vi "Set_coordenadas_estacion.vi"(8 "error in (no error)":errorcluster, 10 "MODO":T1=enum."CONFIG ESTACION", 11 "VISA SESSION":refnum<visa-resource-name>) -> (0 "error out":errorcluster, 3 "Coordenadas_estacion 2":T2)   [LabVIEW 2019]
uses:
  Type_defs/Coordenadas_estacion.ctl
  Type_defs/state_coordenadas.ctl
  LABVIEW_ROBOT_MASTER/Type_defs/TAREAS_ROBOT.ctl
  <vilib>/Utility/error.llb/Error Cluster From Error Code.vi
  <vilib>/ErrorRing/Error Ring.xnode
panel:
  in  "Tab Control":enum32{"Page 1", "Page 2"}(tab)
  in  "EXIT":bool
  in  "CONTINUAR":bool
  in  "Set coordenadas bandejas":bool
  out "COORDENADAS ESTACION DE TRABAJO":T2
  out "Estado FSM":T3
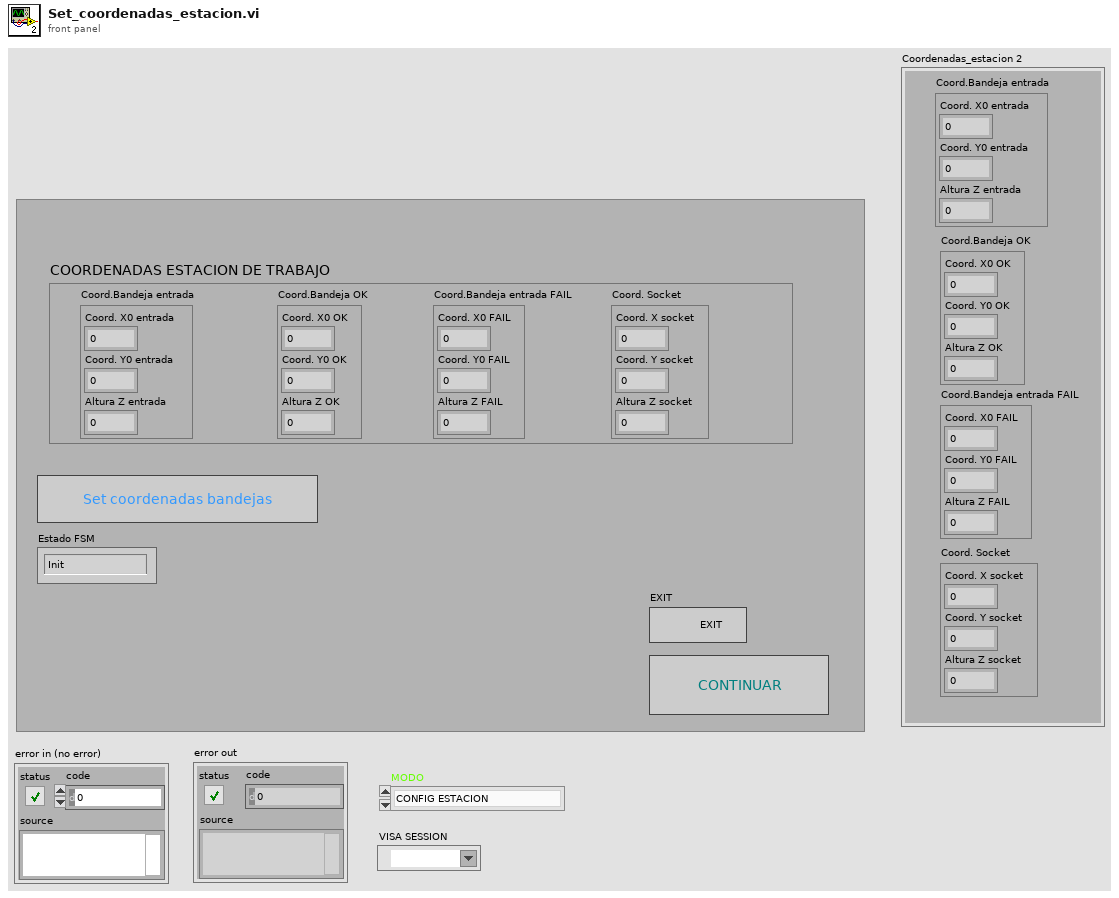
[diagram p1: front panel]
types:
  T1 = typedef "TAREAS_ROBOT.ctl" = enum16{"NINGUNA", "TEST ASICS", "AJUSTE CAM", "MOVER ASICS", "MOVIMIENTO MANUAL", "LEER QR", "CONFIG ESTACION"}
  T2 = typedef "Coordenadas_estacion.ctl" = cluster{"Coord.Bandeja entrada":cluster{"Coord. X0 entrada":u32, "Coord. Y0 entrada ":u32, "Altura Z entrada":u32}, "Coord.Bandeja OK":cluster{"Coord. X0 OK":u32, "Coord. Y0 OK":u32, "Altura Z OK":u32}, "Coord.Bandeja entrada FAIL":cluster{"Coord. X0 FAIL":u32, "Coord. Y0 FAIL":u32, "Altura Z FAIL":u32}, "Coord. Socket":cluster{"Coord. X socket":u32, "Coord. Y socket":u32, "Altura Z socket":u32}}
  T3 = typedef "state_coordenadas.ctl" = enum16{"Init", "Evento", "Vi movimiento manual", "Check values", "Error", "Continuar", "Exit"}
  T4 = enum8{"Enabled", "Disabled", "Disabled and Grayed Out"}
  T5 = cluster{"Coord. X socket":u32, "Coord. Y socket":u32, "Altura Z socket":u32}[]
  T6 = cluster{"Coord. X socket":bool, "Coord. Y socket":bool, "Altura Z socket":bool}
  T7 = cluster{"Coord. X0 entrada":u32, "Coord. Y0 entrada ":u32, "Altura Z entrada":u32}
  T8 = cluster{"Coord. X0 OK":u32, "Coord. Y0 OK":u32, "Altura Z OK":u32}
  T9 = cluster{"Coord. X0 FAIL":u32, "Coord. Y0 FAIL":u32, "Altura Z FAIL":u32}
  T10 = cluster{"Coord. X0 entrada":bool, "Coord. Y0 entrada ":bool, "Altura Z entrada":bool}
  T11 = cluster{"Coord. X0 OK":bool, "Coord. Y0 OK":bool, "Altura Z OK":bool}
  T12 = cluster{"Coord. X0 FAIL":bool, "Coord. Y0 FAIL":bool, "Altura Z FAIL":bool}
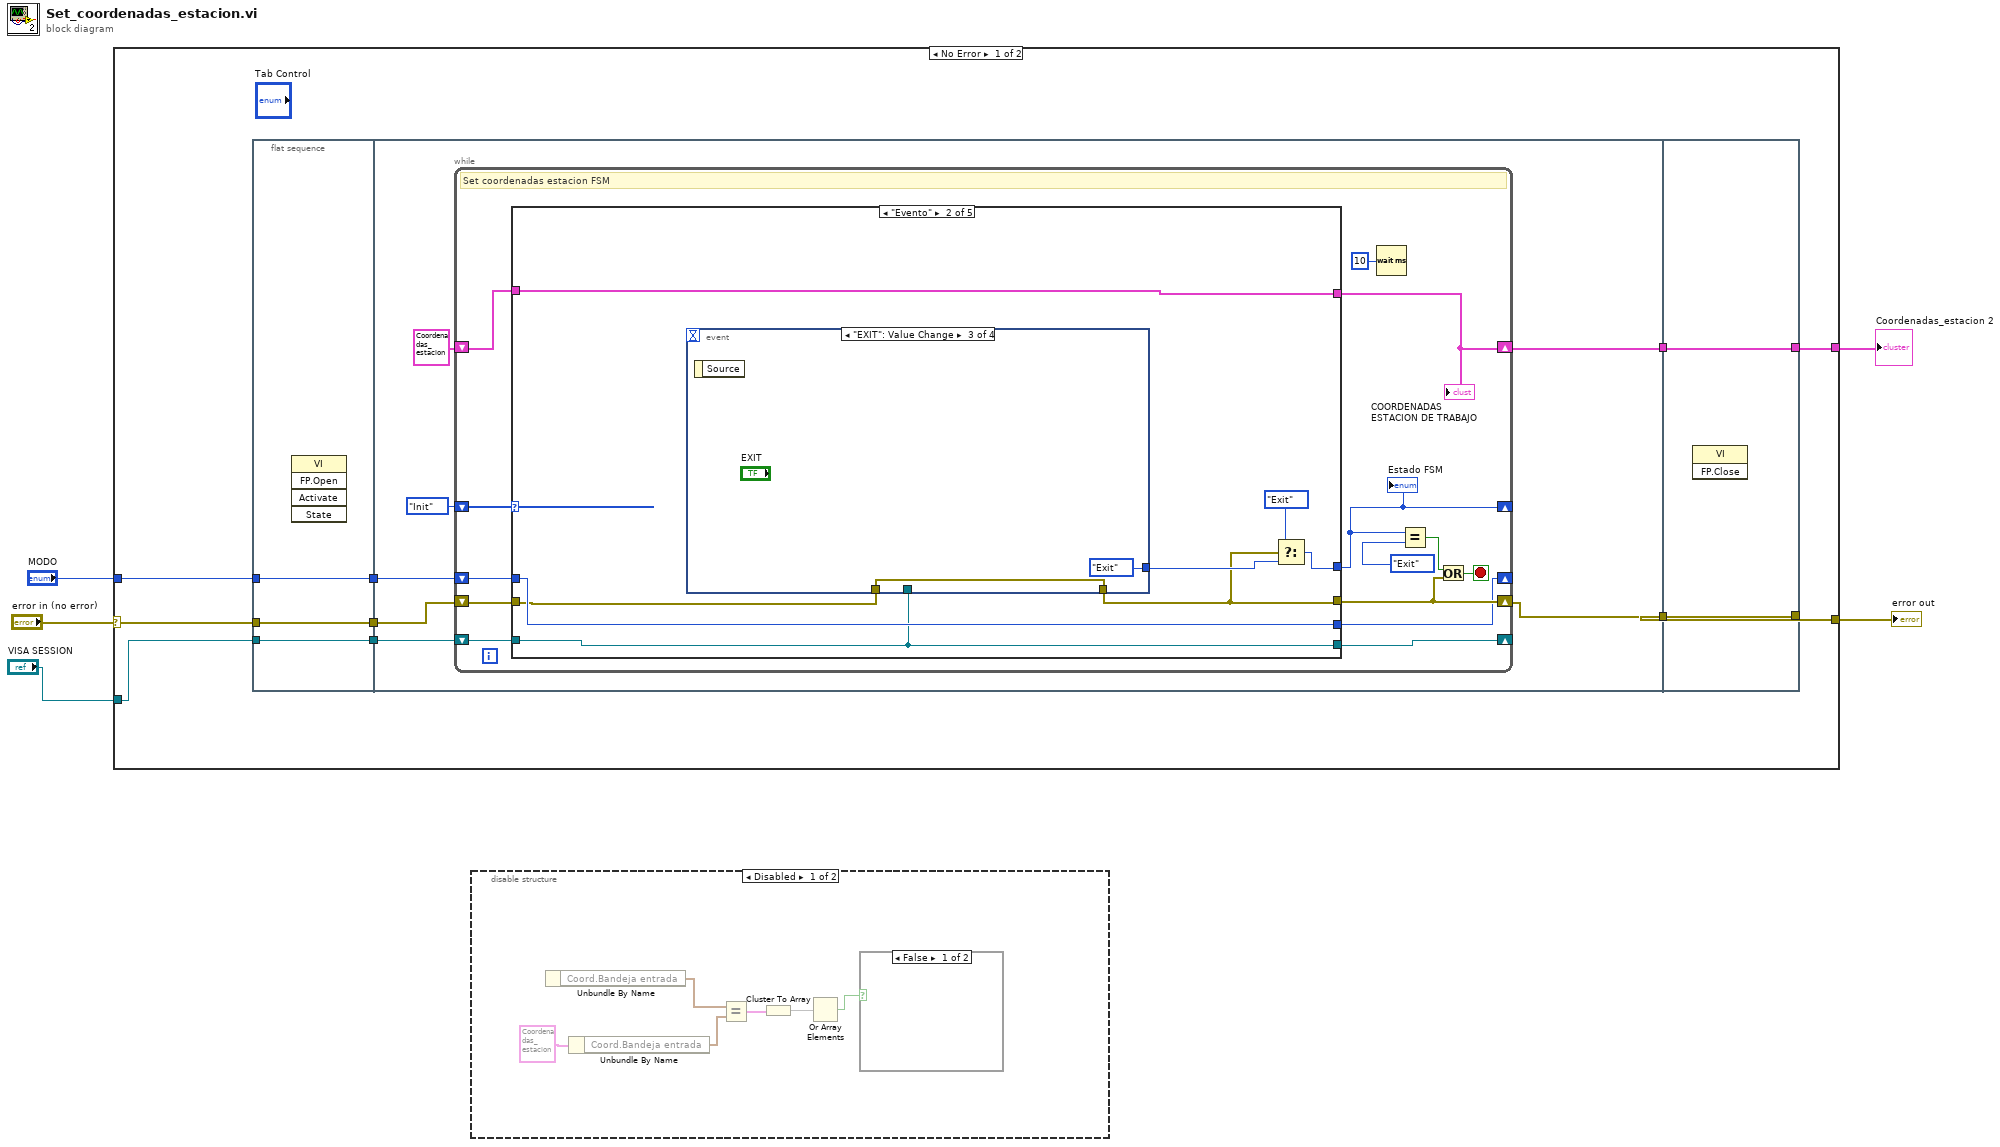
[diagram p0: block diagram]
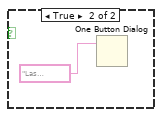
[diagram p2: hidden frame]
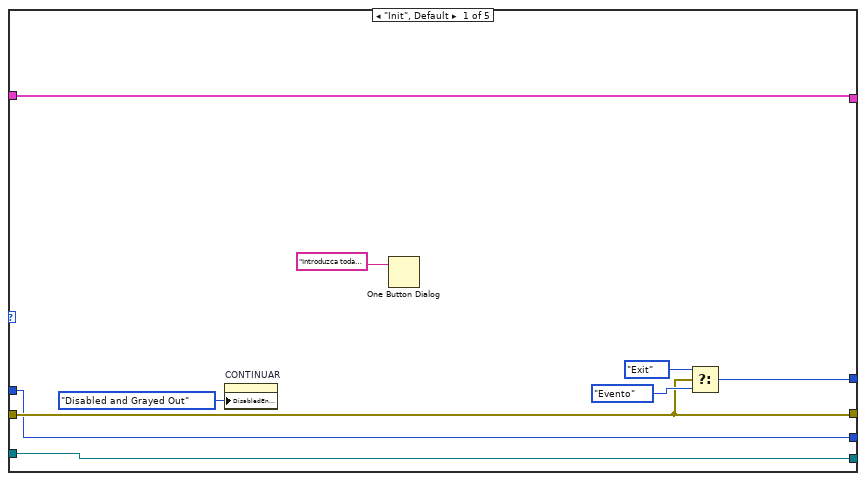
[diagram p4: hidden frame]
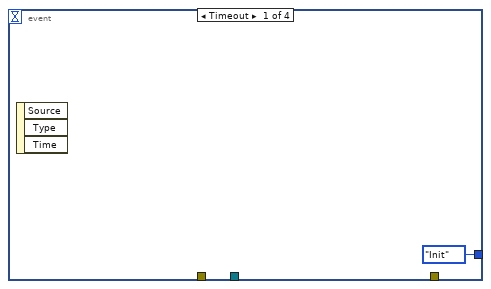
[diagram p5: hidden frame]
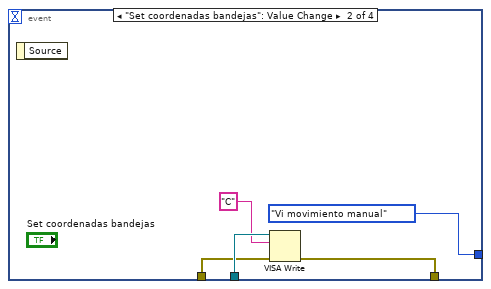
[diagram p6: hidden frame]
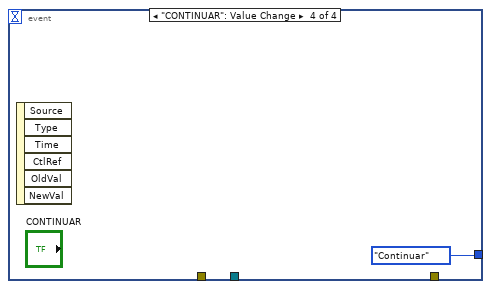
[diagram p7: hidden frame]
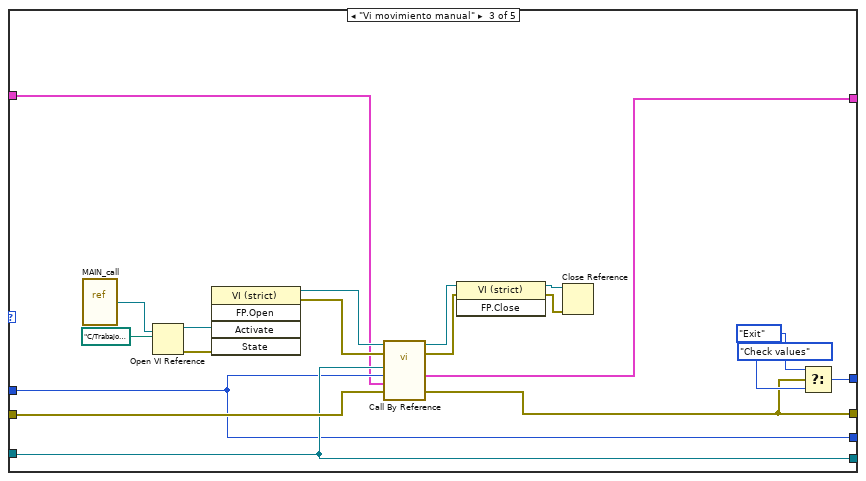
[diagram p8: hidden frame]
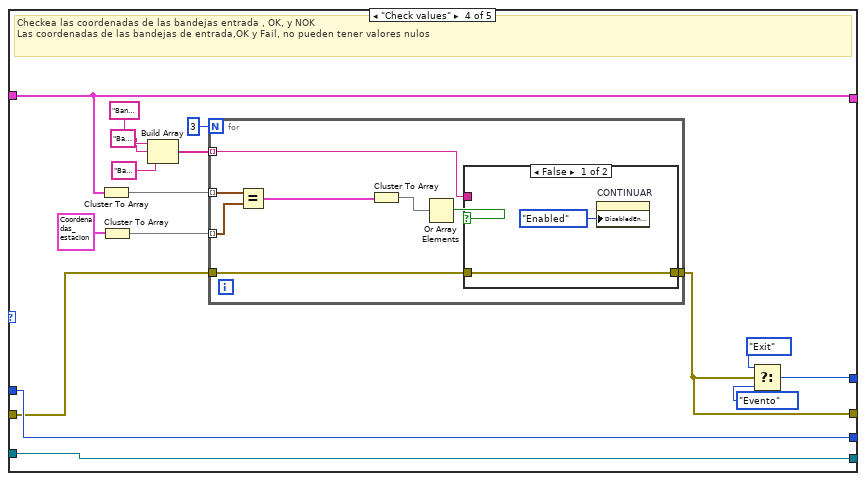
[diagram p9: hidden frame]
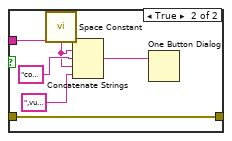
[diagram p10: hidden frame]
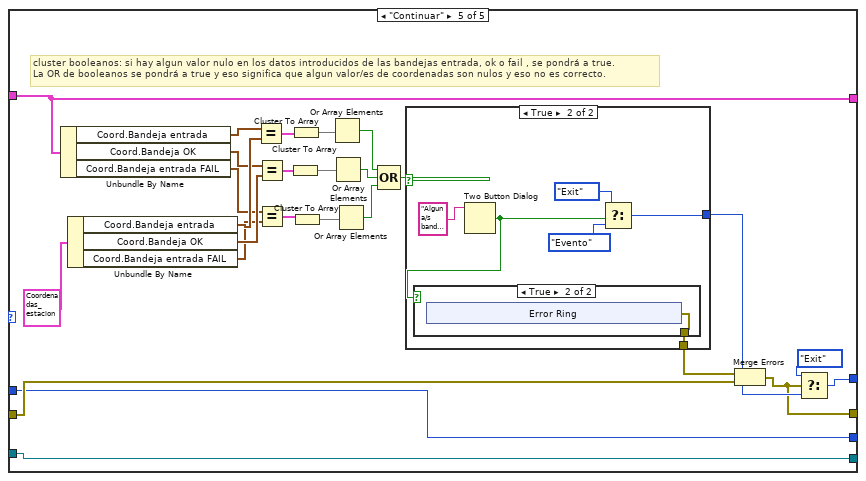
[diagram p11: hidden frame]
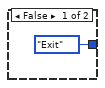
[diagram p12: hidden frame]
diagram:
  n1 = case shown="No Error" "error in (no error)" {
    selector: "error in (no error)" -> [w13 w158]
    tunnel: [w12 w158] -> w4
    tunnel: [w10 _] -> w3
    tunnel: "VISA SESSION" -> [w9 _]
    tunnel: "MODO" -> [w7 _]
    frame No Error {
      n2 = flat-sequence {
        tunnel: w13 -> [w18]
        tunnel: [w18] -> w15
        tunnel: w9 -> [w17]
        tunnel: [w17] -> w8
        tunnel: w7 -> [w16]
        tunnel: [w16] -> w6
        tunnel: w15 -> [w24]
        tunnel: [w19] -> w14
        tunnel: [w22] -> w11
        tunnel: w8 -> [w21]
        tunnel: w6 -> [w20]
        tunnel: w14 -> [w157]
        tunnel: [w157] -> w12
        tunnel: w11 -> [w156]
        tunnel: [w156] -> w10
        frame #0 {
          n3 = invoke class="VI" method="FP.Open"() -> ()  [unwired: 5 in, 5 out]
        }
        frame #1 {
          n4 = while {
            shift-right: [w34] -> _
            shift-left: state_coordenadas."Init" ("Enum") -> [w39]
            shift-right: [w31] -> w19
            shift-left: w24 -> [w37]
            shift-right: [w35] -> w22
            shift-left: T2 {"Coord.Bandeja entrada"={"Coord. X0 entrada"=0, "Coord. Y0 entrada "=0, "Altura Z entrada"=0}, "Coord.Bandeja OK"={"Coord. X0 OK"=0, "Coord. Y0 OK"=0, "Altura Z OK"=0}, "Coord.Bandeja entrada FAIL"={"Coord. X0 FAIL"=0, "Coord. Y0 FAIL"=0, "Altura Z FAIL"=0}, "Coord. Socket"={"Coord. X socket"=0, "Coord. Y socket"=0, "Altura Z socket"=0}} ("Coordenadas_estacion") -> [w36]
            shift-right: [w28] -> _
            shift-left: w21 -> [w29]
            shift-right: [w26] -> _
            shift-left: w20 -> [w27]
            stop <- w30 stop-if-true
            # "Set coordenadas estacion FSM"
            n5 = case shown="\"Evento\"" w39 {
              tunnel: w37 -> [w44 w50 w73 w87 w123]
              tunnel: [w44 w49 w72 w86 w118] -> w31
              tunnel: w36 -> [w43 w53 w66 w93 w142]
              tunnel: [w43 w53 w67 w93 w142] -> w35
              tunnel: [w45 w54 w81 w97 w120] -> w34
              tunnel: w29 -> [w42 w51 w69 w100 w119]
              tunnel: [w42 w51 w69 w100 w119] -> w28
              tunnel: w27 -> [w41 w52 w68 w96 w117]
              tunnel: [w41 w52 w68 w96 w117] -> w26
              frame "Init", Default {
                n6 = property on="CONTINUAR" class="Bool"("DisabledEnum"=T4."Disabled and Grayed Out" ("Disabled")) -> ()  [unwired: 2 in, 2 out]
                n7 = One Button Dialog(message="Introduzca todas las coordenadas para configurar la estación") -> ()  [unwired: 1 in, 1 out]
                n8 = Select(t=state_coordenadas."Exit", s=w44, f=state_coordenadas."Evento" ("Enum")) -> (s? t:f=w45:T3)
              }
              frame "Evento" {
                n9 = event shown="[2] \"EXIT\": Value Change" {
                  selector: _ -> [_ _ _ _]
                  dyn-events: _ -> [_ _ _ _]
                  timeout: _ -> [_ _ _ _]
                  tunnel: [state_coordenadas."Init" ("Enum") state_coordenadas."Vi movimiento manual" ("Enum") state_coordenadas."Exit" ("Enum") state_coordenadas."Continuar" ("Enum")] -> w56
                  tunnel: w51 -> [_ w61 _ _]
                  tunnel: w50 -> [_ w59 w64 _]
                  tunnel: [_ w58 w64 _] -> w49
                  event Timeout {
                    n10 = event-data() -> ()  [unwired: 1 in, 3 out]
                  }
                  event "Set coordenadas bandejas": Value Change {
                    n11 = event-data() -> ()  [unwired: 1 in, 1 out]
                    n12 = VISA Write(VISA resource name=w61, write buffer="C", error in (no error)=w59) -> (error out=w58:errorcluster)  [unwired: 2 out]
                  }
                  event "EXIT": Value Change {
                    n13 = event-data() -> ()  [unwired: 1 in, 1 out]
                  }
                  event "CONTINUAR": Value Change {
                    n14 = event-data() -> ()  [unwired: 1 in, 6 out]
                  }
                }
                n15 = Select(t=state_coordenadas."Exit", s=w49, f=w56) -> (s? t:f=w54:T3)
              }
              frame "Vi movimiento manual" {
                n16 = vi-ref "MAIN_call.vi"() -> (w84:refnum<vi>)
                n17 = Open VI Reference(type specifier VI Refnum (for type only)=w84, vi path=path "C:/Trabajo_Robot/TFG_ROBOT/CONTROL_ROBOT/LVPROJ_MOVIMIENTO_CABEZAL/LABVIEW_MOVIMIENTO/MOVIMIENTO CABEZAL/MAIN_call.vi") -> (vi reference=w79:refnum<vi>, error out=w77:errorcluster)  [unwired: 4 in]
                n18 = invoke class="VI (strict)" method="FP.Open"(reference=w79, error in=w77) -> (reference out=w78:refnum<vi>, error out=w76:errorcluster)  [unwired: 3 in, 3 out]
                n19 = call-by-ref "?"(reference=w78, error in=w76, "error IO"=w73, "Coordenadas_estacion_input"=w66, "Modo"=w68, "VISA SESSION"=w69) -> (reference out=w75:refnum<vi>, error out=w74:errorcluster, 0:"error out"=w72:errorcluster, "Coordenadas_estacion_outpu"=w67:T2)  [unwired: 6 in]
                n20 = invoke class="VI (strict)" method="FP.Close"(reference=w75, error in=w74) -> (reference out=w71:refnum<vi>, error out=w70:errorcluster)  [unwired: 1 in, 1 out]
                n21 = Close Reference(reference=w71, error in (no error)=w70) -> ()  [unwired: 1 out]
                n22 = Select(t=state_coordenadas."Exit", s=w72, f=state_coordenadas."Check values" ("Enum")) -> (s? t:f=w81:T3)
              }
              frame "Check values" {
                # "Checkea las coordenadas de las bandejas entrada , OK, y NOK\nLas coordenadas de las bandejas de entrada,OK y Fail, no pueden tener valores nulos"
                n23 = Cluster To Array(cluster=w93) -> (array=w85:T5)
                n24 = Cluster To Array(cluster=T2 {"Coord.Bandeja entrada"={"Coord. X0 entrada"=0, "Coord. Y0 entrada "=0, "Altura Z entrada"=0}, "Coord.Bandeja OK"={"Coord. X0 OK"=0, "Coord. Y0 OK"=0, "Altura Z OK"=0}, "Coord.Bandeja entrada FAIL"={"Coord. X0 FAIL"=0, "Coord. Y0 FAIL"=0, "Altura Z FAIL"=0}, "Coord. Socket"={"Coord. X socket"=0, "Coord. Y socket"=0, "Altura Z socket"=0}} ("Coordenadas_estacion")) -> (array=w94:T5)
                n25 = Build Array("Bandeja entrada", "Bandeja OK" ("element"), "Bandeja NOK" ("element")) -> (w89:string[])
                n26 = for {
                  N: 3 -> [_]
                  tunnel: w85 -> [w108] mode=indexing
                  tunnel: w94 -> [w107] mode=indexing
                  tunnel: w89 -> [w103] mode=indexing
                  tunnel: w87 -> [w102]
                  tunnel: [w101] -> w86
                  n27 = Equal?(x=w108, y=w107) -> (x = y?=w106:T6)
                  n28 = Cluster To Array(cluster=w106) -> (array=w105:bool[])
                  n29 = Or Array Elements(Boolean array=w105) -> (logical OR=w104:bool)
                  n30 = case shown="False" w104 {
                    tunnel: w103 -> [_ w116]
                    tunnel: w102 -> [w110 w111]
                    tunnel: [w110 w111] -> w101
                    frame False {
                      n31 = property on="CONTINUAR" class="Bool"("DisabledEnum"=T4."Enabled" ("Disabled")) -> ()  [unwired: 2 in, 2 out]
                    }
                    frame True {
                      n32 = call <vilib>:"Space Constant.vi"() -> ("String"=w113:string)
                      n33 = Concatenate Strings(w116, w113, "con alguna/s coordendanula", w113, ",vuelva a adquirir coordenada.") -> (w114:string)
                      n34 = One Button Dialog(message=w114) -> ()  [unwired: 1 in, 1 out]
                    }
                  }
                }
                n35 = Select(t=state_coordenadas."Exit" ("y"), s=w86, f=state_coordenadas."Evento") -> (s? t:f=w97:T3)
              }
              frame "Continuar" {
                # "cluster booleanos: si hay algun valor nulo en los datos introducidos de las bandejas entrada, ok o fail , se pondrá a true.\nLa OR de booleanos se pondrá a true y eso significa que algun valor/es de coordenadas son nulos y eso no es correcto."
                n36 = Unbundle By Name(w142) -> ("Coord.Bandeja entrada"=w141:T7, "Coord.Bandeja OK"=w138:T8, "Coord.Bandeja entrada FAIL"=w135:T9)
                n37 = Unbundle By Name(T2 {"Coord.Bandeja entrada"={"Coord. X0 entrada"=0, "Coord. Y0 entrada "=0, "Altura Z entrada"=0}, "Coord.Bandeja OK"={"Coord. X0 OK"=0, "Coord. Y0 OK"=0, "Altura Z OK"=0}, "Coord.Bandeja entrada FAIL"={"Coord. X0 FAIL"=0, "Coord. Y0 FAIL"=0, "Altura Z FAIL"=0}, "Coord. Socket"={"Coord. X socket"=0, "Coord. Y socket"=0, "Altura Z socket"=0}} ("Coordenadas_estacion")) -> ("Coord.Bandeja entrada"=w139:T7, "Coord.Bandeja OK"=w137:T8, "Coord.Bandeja entrada FAIL"=w136:T9)
                n38 = Equal?(x=w141, y=w139) -> (x = y?=w134:T10)
                n39 = Equal?(x=w138, y=w137) -> (x = y?=w132:T11)
                n40 = Equal?(x=w135, y=w136) -> (x = y?=w131:T12)
                n41 = Cluster To Array(cluster=w132) -> (array=w130:bool[])
                n42 = Cluster To Array(cluster=w134) -> (array=w133:bool[])
                n43 = Cluster To Array(cluster=w131) -> (array=w129:bool[])
                n44 = Or Array Elements(Boolean array=w133) -> (logical OR=w128:bool)
                n45 = Or Array Elements(Boolean array=w130) -> (logical OR=w127:bool)
                n46 = Or Array Elements(Boolean array=w129) -> (logical OR=w126:bool)
                n47 = Compound Arithmetic op=OR(w128, w127, w126) -> (w125:bool)
                n48 = case shown="True" w125 {
                  tunnel: [_ w145] -> w124
                  tunnel: [state_coordenadas."Exit" ("y") w144] -> w122
                  frame False {
                  }
                  frame True {
                    n49 = Two Button Dialog(message="Alguna/s bandeja de entrada,OK, y FAIL tienen valores nulos.\n¿Desea continuar?") -> (T button?=w146:bool)  [unwired: 2 in]
                    n50 = case shown="True" w146 {
                      tunnel: [_ w150] -> w145
                      frame False {
                      }
                      frame True {
                        n51 = xnode "Error Ring"() -> ("error out"=w150:errorcluster)
                      }
                    }
                    n52 = Select(t=state_coordenadas."Exit" ("y"), s=w146, f=state_coordenadas."Evento" ("y")) -> (s? t:f=w144:T3)
                  }
                }
                n53 = Merge Errors(w124, w123) -> (w118:errorcluster)
                n54 = Select(t=state_coordenadas."Exit", s=w118, f=w122) -> (s? t:f=w120:T3)
              }
            }
            "COORDENADAS ESTACION DE TRABAJO" <- w35
            "Estado FSM" <- w34
            n55 = Wait (ms)(milliseconds to wait=u32 10) -> ()  [unwired: 1 out]
            n56 = Equal?(x=w34, y=state_coordenadas."Exit") -> (x = y?=w32:bool)
            n57 = Or(x=w32, y=w31) -> (x .or. y?=w30:bool)
          }
        }
        frame #2 {
          n58 = invoke class="VI" method="FP.Close"() -> ()  [unwired: 3 in, 3 out]
        }
      }
    }
    frame Error {
    }
  }
  "error out" <- w4
  "Coordenadas_estacion 2" <- w3
  n59 = disable-structure shown="Disabled" {
    frame Disabled {
      n60 = Unbundle By Name() -> ("Coord.Bandeja entrada"=w164:T7)  [unwired: 1 in]
      n61 = Unbundle By Name(T2 {"Coord.Bandeja entrada"={"Coord. X0 entrada"=0, "Coord. Y0 entrada "=0, "Altura Z entrada"=0}, "Coord.Bandeja OK"={"Coord. X0 OK"=0, "Coord. Y0 OK"=0, "Altura Z OK"=0}, "Coord.Bandeja entrada FAIL"={"Coord. X0 FAIL"=0, "Coord. Y0 FAIL"=0, "Altura Z FAIL"=0}, "Coord. Socket"={"Coord. X socket"=0, "Coord. Y socket"=0, "Altura Z socket"=0}} ("Coordenadas_estacion")) -> ("Coord.Bandeja entrada"=w162:T7)
      n62 = Equal?(x=w164, y=w162) -> (x = y?=w161:T10)
      n63 = Cluster To Array(cluster=w161) -> (array=w160:bool[])
      n64 = Or Array Elements(Boolean array=w160) -> (logical OR=w159:bool)
      n65 = case shown="False" w159 {
        frame False {
        }
        frame True {
          n66 = One Button Dialog(message="Las coordenadas introducidas para la bandeja de entrada no pueden ser cero ") -> ()  [unwired: 1 in, 1 out]
        }
      }
    }
    frame Enabled {
    }
  }
